vi "Query Measurement Multiplier.vi"(8 "error in (no error)":errorcluster {"code" format="%.0x"}, 9 "RetValBufferSize":i32=2048, 11 "instrument handle":refnum<k15>) -> (0 "error out":errorcluster {"code" format="%.0x"}, 1 "RetValActualSize":i32, 2 "RetVal":i32[](array[numeric]), 3 "instrument handle out":refnum<k15>)   [LabVIEW 2021, in "Keysight XSAnVMA.lvlib"]
doc: "Queries the multiplier of Resolution Bandwidth for the measurement integration bandwidth."
uses:
  <instrlib>/Keysight XSAnVMA/Keysight XSAnVMA.lvlib
  KtXSAnVMA_64.dll
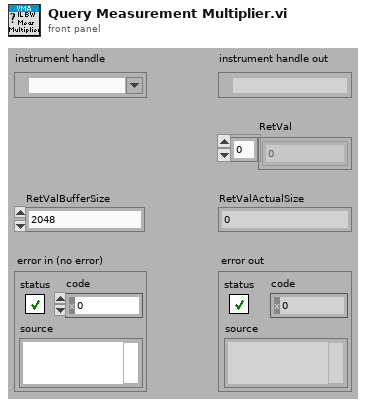
[diagram p1: front panel]
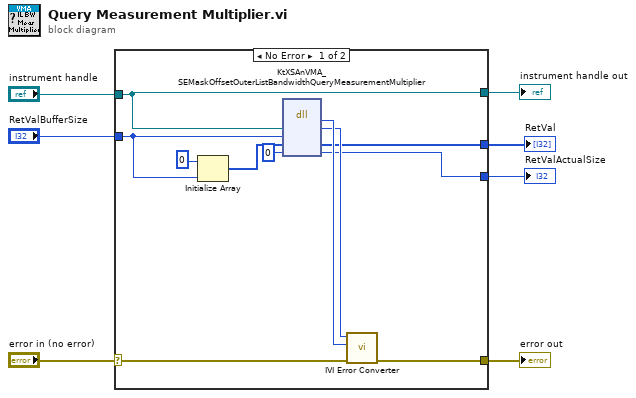
[diagram p0: block diagram]
diagram:
  n1 = case shown="No Error" "error in (no error)" {
    selector: "error in (no error)" -> [w18 w20]
    tunnel: [w17 w20] -> w7
    tunnel: "instrument handle" -> [w15 w19]
    tunnel: "RetValBufferSize" -> [w14 _]
    tunnel: [w9 _] -> w3
    tunnel: [w8 _] -> w2
    tunnel: [w15 w19] -> w1
    frame No Error {
      n2 = Initialize Array(0 ("element"), w14) -> (w13:i32[])
      n3 = dll-call lib="KtXSAnVMA**.dll" fn="KtXSAnVMA_SEMaskOffsetOuterListBandwidthQueryMeasurementMultiplier"("Vi"=w15, "RetValBufferSize"=w14, "RetVal"=w13, "RetValActualSize"=0) -> ("return type"=w11:i32, "Vi"=w10:u32, "RetVal"=w9:u16[], "RetValActualSize"=w8:i32)  [unwired: 4 in, 2 out]
      n4 = call <instrlib>:"IVI Error Converter.vi"("error in (no error)"=w18, "IVI error code (0)"=w11, "instrument handle"=w10) -> ("error out"=w17:errorcluster)  [unwired: 7 in, 1 out]
    }
    frame Error {
    }
  }
  "error out" <- w7
  "instrument handle out" <- w1
  "RetVal" <- w3
  "RetValActualSize" <- w2
